vi "UMLEditor ToolsMenuUpdates.vi"(0 "menu":refnum<k9>, 2 "item":string, 3 "Graph":refnum<class "Graph.lvclass">, 5 "error in (no error)":errorcluster) -> (19 "error out":errorcluster)   [LabVIEW 2020]
doc: "Gets current diagram values"
uses:
  <resource>/Framework/Providers/Open_GDS/UML/Graph_class/Graph.lvclass
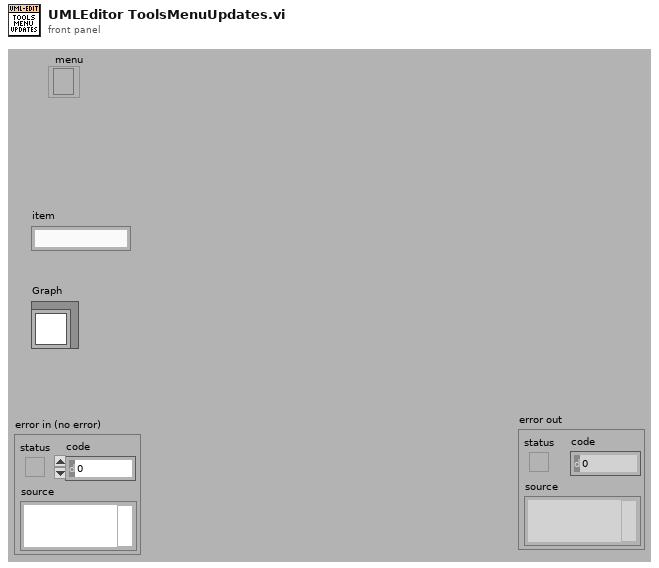
[diagram p1: front panel]
types:
  T1 = cluster{string, string, "short cut out":cluster{"include Shift key?":bool, "include Ctrl key? ":bool, "shortcut key":string}}[]
  T2 = cluster{"include Shift key?":bool, "include Ctrl key? ":bool, "shortcut key":string}
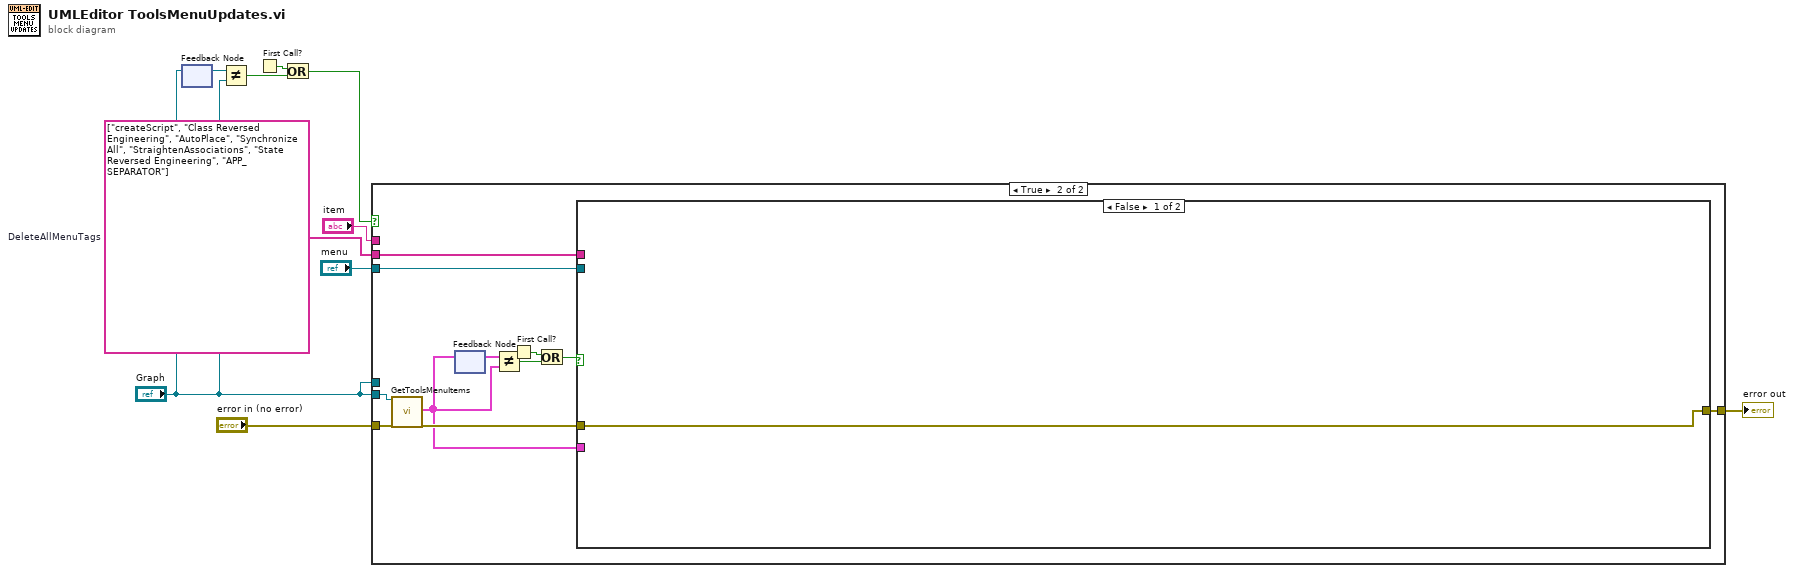
[diagram p0: block diagram]
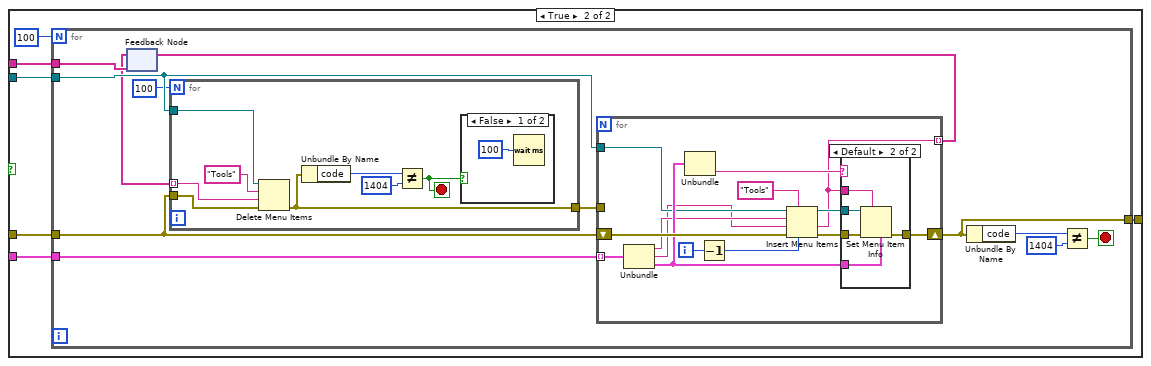
[diagram p3: hidden frame]
diagram:
  w6 = string[] ["createScript", "Class Reversed Engineering", "AutoPlace", "Synchronize All", "StraightenAssociations", "State Reversed Engineering", "APP_SEPARATOR"]  # DeleteAllMenuTags
  n1 = feedback #1() -> (w5:refnum<class "Graph.lvclass">)  [unwired: 1 in]
  n2 = feedback-in #1("Graph") -> ()
  n3 = Not Equal?(x=w5, y="Graph") -> (x != y?=w3:bool)
  n4 = First Call?() -> (First Call?: T/F=w4:bool)
  n5 = Or(x=w4, y=w3) -> (x .or. y?=w2:bool)
  n6 = case shown="True" w2 {
    tunnel: [w11 w22] -> w9
    tunnel: "menu" -> [_ w21]
    tunnel: "Graph" -> [_ _]
    tunnel: "item" -> [_ _]
    tunnel: "error in (no error)" -> [w11 w20]
    tunnel: w6 -> [_ w18]
    tunnel: "Graph" -> [_ w19]
    frame False {
    }
    frame True {
      n7 = call-dynamic "GetToolsMenuItems.vi"("reference in"=w19, "error in (no error)"=w20) -> ("ToolMenuItems"=w13:T1, "error out"=w17:errorcluster)  [unwired: 15 in, 1 out]
      n8 = feedback #2() -> (w14:T1)  [unwired: 1 in]
      n9 = feedback-in #2(w13) -> ()
      n10 = Not Equal?(x=w14, y=w13) -> (x != y?=w16:bool)
      n11 = First Call?() -> (First Call?: T/F=w15:bool)
      n12 = Or(x=w15, y=w16) -> (x .or. y?=w12:bool)
      n13 = case shown="False" w12 {
        tunnel: [w23 w29] -> w22
        tunnel: w21 -> [_ w28]
        tunnel: w18 -> [_ w27]
        tunnel: w17 -> [w23 w26]
        tunnel: w13 -> [_ w24]
        frame False {
        }
        frame True {
          n14 = for {
            N: 100 -> [_]
            tunnel: w28 -> [w41]
            tunnel: w24 -> [w40]
            tunnel: w27 -> [w38]
            tunnel: w26 -> [w34]
            tunnel: [w31] -> w29
            stop <- w30 stop-if-true
            n15 = feedback #3(w38) -> (w37:string[])
            n16 = for {
              N: 100 -> [_]
              tunnel: w41 -> [w49]
              tunnel: w37 -> [w46] mode=indexing
              tunnel: w34 -> [w47]
              tunnel: [w45] -> w36
              stop <- w42 stop-if-true
              n17 = Delete Menu Items(6:w47, 7:w46, 8:"Tools" ("item tag"), 9:w49) -> (0:w45:errorcluster)  [unwired: 1 out]
              n18 = Unbundle By Name(w45) -> ("code"=w44:i32)
              n19 = Not Equal?(x=w44, y=1404) -> (x != y?=w42:bool)
              n20 = case shown="False" w42 {
                frame False {
                  n21 = Wait (ms)(milliseconds to wait=u32 100) -> ()  [unwired: 1 out]
                }
                frame True {
                }
              }
            }
            n22 = for {
              tunnel: w40 -> [w62] mode=indexing
              shift-right: [w57] -> w31
              shift-left: w34 -> [w61]
              tunnel: w41 -> [w58]
              tunnel: [w51] -> w39 mode=indexing
              tunnel: w36 -> [_]
              i -> [w55]
              n23 = Unbundle(w62) -> (w59:string, w52:string, "short cut out"=w60:T2)
              n24 = Unbundle(w60) -> ("shortcut key"=w53:string)  [unwired: 2 out]
              n25 = Decrement(x=w55) -> (x-1=w54:i32)
              n26 = Insert Menu Items(4:w54, 5:"Tools" ("menu tag"), 6:w61, 7:w52, 8:w59, 9:w58) -> (0:w56:errorcluster, 1:w51:string, 3:w63:refnum<k9>)
              n27 = case shown="Default" w53 {
                tunnel: w63 -> [_ w70]
                tunnel: w60 -> [_ w66]
                tunnel: w51 -> [_ w69]
                tunnel: [w65 w68] -> w57
                tunnel: w56 -> [w65 w67]
                frame "" {
                }
                frame Default {
                  n28 = Set Menu Item Info(4:w66, 7:w69, 8:w67, 11:w70) -> (0:w68:errorcluster)  [unwired: 4 out]
                }
              }
            }
            n29 = feedback-in #3(w39) -> ()
            n30 = Unbundle By Name(w31) -> ("code"=w32:i32)
            n31 = Not Equal?(x=w32, y=1404) -> (x != y?=w30:bool)
          }
        }
      }
    }
  }
  "error out" <- w9
